vi "Polynomial Roots (DBL).vi"(10 "option":u16(ring)=1 items=["General", "Simple Classification", "Refinement", "Advanced Refinement"], 11 "P(x)":dbl[](array[numeric])) -> (0 "error":i32, 3 "Roots":cdb[](array[numeric]))   [LabVIEW 2010, in "NI_AALPro.lvlib"]
doc: "Finds the roots of polynomial <B>P(x)</B>. This VI removes leading coefficients of the polynomial that are equal to zero. Wire data to the <B>P(x)</B> input to determine the polymorphic instance to use or manually select the instance."
uses:
  NI_AALPro.lvlib
  Remove Zero Coefficients (DBL).vi
  lvanlys.dll
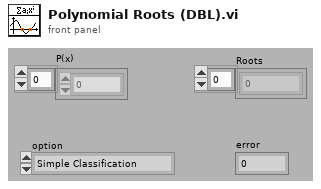
[diagram p1: front panel]
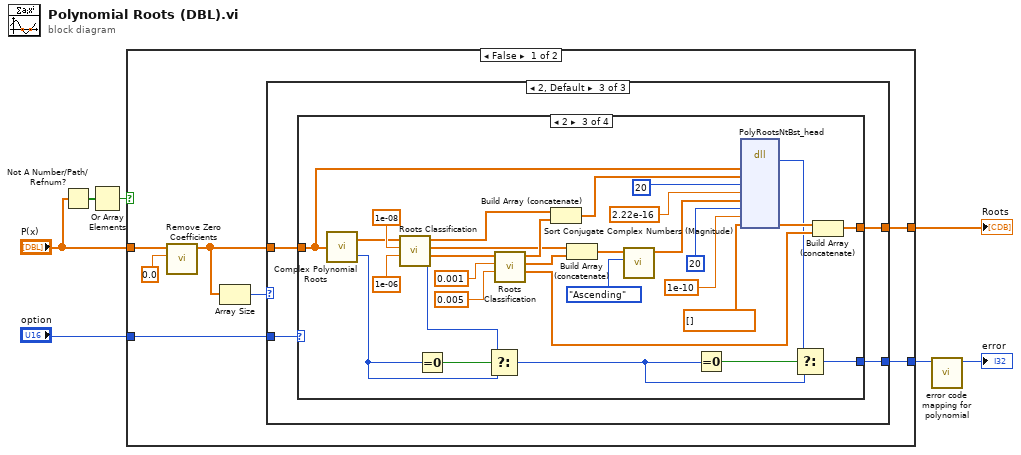
[diagram p0: block diagram]
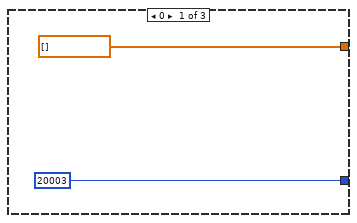
[diagram p2: hidden frame]
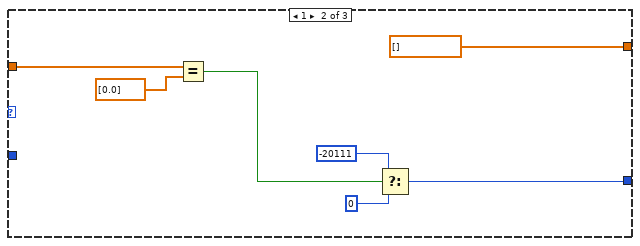
[diagram p3: hidden frame]
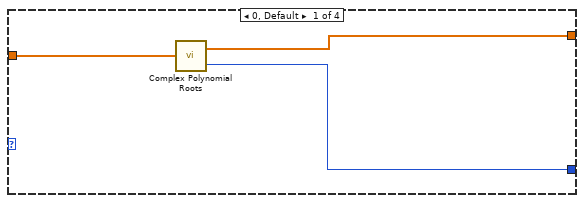
[diagram p4: hidden frame]
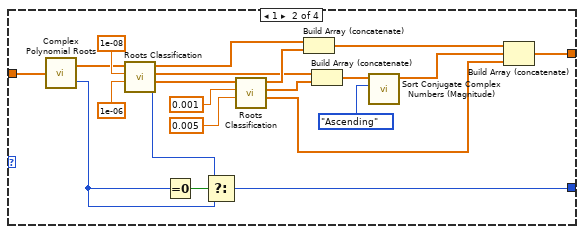
[diagram p5: hidden frame]
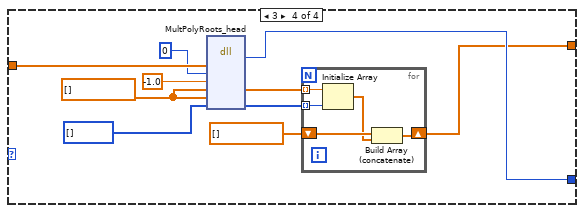
[diagram p6: hidden frame]
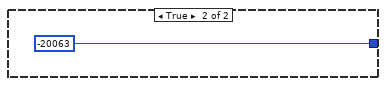
[diagram p7: hidden frame]
diagram:
  n1 = Not A Number/Path/Refnum?(number/path/refnum="P(x)") -> (NaN/Path/Refnum?=w2:bool[])
  n2 = Or Array Elements(Boolean array=w2) -> (logical OR=w1:bool)
  n3 = case shown="False" w1 {
    tunnel: [w14 _] -> w7
    tunnel: "option" -> [w12 _]
    tunnel: [w11 -20063 ("error")] -> w5
    tunnel: "P(x)" -> [w9 _]
    frame False {
      n4 = call-poly "Remove Zero Coefficients.vi"("threshold"=0.0, "P(x) In"=w9) -> ("P(x) Out"=w8:dbl[])  [unwired: 1 in, 8 out]
      n5 = Array Size(array=w8) -> (size(s)=w13:i32)
      n6 = case shown="2, Default" w13 {
        tunnel: w8 -> [_ w23 w24]
        tunnel: [20003 ("empty array") w18 w27] -> w11
        tunnel: [cdb[] [] cdb[] [] ("Polynomial Roots") w26] -> w14
        tunnel: w12 -> [_ _ w25]
        frame 0 {
        }
        frame 1 {
          n7 = Equal?(x=w23, y=dbl[] [0.0]) -> (x = y?=w20:bool)
          n8 = Select(t=-20111, s=w20, f=0) -> (s? t:f=w18:i32)
        }
        frame 2, Default {
          n9 = case shown="2" w25 {
            tunnel: w24 -> [w28 w31 w56 w91]
            tunnel: [w29 w33 w52 w89] -> w27
            tunnel: [w30 w41 w71 w88] -> w26
            frame 0, Default {
              n10 = call "Complex Polynomial Roots.vi"("Polynomial"=w28) -> ("Polynomial Roots"=w30:cdb[], "error"=w29:i32)
            }
            frame 1 {
              n11 = call "Complex Polynomial Roots.vi"("Polynomial"=w31) -> ("Polynomial Roots"=w39:cdb[], "error"=w34:i32)
              n12 = call "Roots Classification.vi"("tolerance for conjugate pair"=1e-06 ("threshold"), "tolerance for real roots"=1e-08 ("threshold"), "Roots"=w39) -> ("error"=w32:i32, "Pure Complex Roots"=w48:cdb[], "Complex Pair Roots"=w44:cdb[], "Real Roots"=w49:dbl[])  [unwired: 5 out]
              n13 = Equal To 0?(x=w34) -> (x = 0?=w35:bool)
              n14 = Select(t=w32, s=w35, f=w34) -> (s? t:f=w33:i32)
              n15 = call "Roots Classification.vi"("tolerance for conjugate pair"=0.005 ("tolerance for real roots"), "tolerance for real roots"=0.001, "Roots"=w48) -> ("Pure Complex Roots"=w40:cdb[], "Complex Pair Roots"=w43:cdb[], "Real Roots"=w45:dbl[])  [unwired: 6 out]
              n16 = Build Array (concatenate)(w49, w45) -> (w38:dbl[])
              n17 = Build Array (concatenate)(w44, w43) -> (w42:cdb[])
              n18 = call "Sort Conjugate Complex Numbers (Magnitude).vi"("Order"=enum16{"Ascending", "Descending"}."Ascending", "Conjugate Complex Numbers"=w42) -> ("Sorted Conjugate Complex Numbers"=w37:cdb[])  [unwired: 9 out]
              n19 = Build Array (concatenate)(w38, w37, w40) -> (w41:cdb[])
            }
            frame 2 {
              n20 = call "Complex Polynomial Roots.vi"("Polynomial"=w56) -> ("Polynomial Roots"=w69:cdb[], "error"=w65:i32)
              n21 = call "Roots Classification.vi"("tolerance for conjugate pair"=1e-06 ("threshold"), "tolerance for real roots"=1e-08 ("threshold"), "Roots"=w69) -> ("error"=w66:i32, "Pure Complex Roots"=w78:cdb[], "Complex Pair Roots"=w74:cdb[], "Real Roots"=w79:dbl[])  [unwired: 5 out]
              n22 = Equal To 0?(x=w65) -> (x = 0?=w67:bool)
              n23 = Select(t=w66, s=w67, f=w65) -> (s? t:f=w53:i32)
              n24 = call "Roots Classification.vi"("tolerance for conjugate pair"=0.005 ("tolerance for real roots"), "tolerance for real roots"=0.001, "Roots"=w78) -> ("Pure Complex Roots"=w70:cdb[], "Complex Pair Roots"=w73:cdb[], "Real Roots"=w75:dbl[])  [unwired: 6 out]
              n25 = Build Array (concatenate)(w79, w75) -> (w64:dbl[])
              n26 = Build Array (concatenate)(w74, w73) -> (w72:cdb[])
              n27 = call "Sort Conjugate Complex Numbers (Magnitude).vi"("Order"=enum16{"Ascending", "Descending"}."Ascending", "Conjugate Complex Numbers"=w72) -> ("Sorted Conjugate Complex Numbers"=w57:cdb[])  [unwired: 9 out]
              n28 = Equal To 0?(x=w53) -> (x = 0?=w55:bool)
              n29 = dll-call lib="C:/Program Files/National Instruments/LabVIEW 2010/resource/lvanlys.*" fn="PolyRootsNtBst_head"("poly"=w56, "FlRootsIn"=w64, "FlMaxIter"=20, "FlTol"=2.22e-16 ("2^x"), "CxRootsIn"=w57, "CxMaxIter"=20 ("FlMaxIter"), "CxTol"=1e-10 ("2^x"), "RootsOut"=cdb[] [] ("Roots")) -> ("return type"=w54:i32, "RootsOut"=w58:cdb[])  [unwired: 10 in, 2 out]
              n30 = Select(t=w54, s=w55, f=w53) -> (s? t:f=w52:i32)
              n31 = Build Array (concatenate)(w58, w70) -> (w71:cdb[])
            }
            frame 3 {
              w85 = cdb[] []
              n32 = dll-call lib="C:/Program Files/National Instruments/LabVIEW 2010/resource/lvanlys.*" fn="MultPolyRoots_head"("pH"=w91, "alg2"=0, "tol"=-1.0, "appRootH"=w85, "rootH"=w85, "multH"=i32[] []) -> ("return type"=w89:i32, "appRootH"=w82:cdb[], "multH"=w86:i32[])  [unwired: 6 in, 3 out]
              n33 = for {
                tunnel: w82 -> [w96] mode=indexing
                tunnel: w86 -> [w95] mode=indexing
                shift-right: [w92] -> w88
                shift-left: cdb[] [] -> [w94]
                n34 = Initialize Array(w96, w95) -> (w93:cdb[])
                n35 = Build Array (concatenate)(w94, w93) -> (w92:cdb[])
              }
            }
          }
        }
      }
    }
    frame True {
    }
  }
  "Roots" <- w7
  n36 = call "error code mapping for polynomial.vi"("error in"=w5) -> ("error out"=→"error":i32)  [unwired: 10 out]
